vi "tfH12.vi"(0 "Resp1":dbl[](array[numeric]), 2 "采样率":i32, 4 "Resp2":dbl[](array[numeric])) -> (5 "ff":dbl[](array[numeric]), 6 "H12":cdb[](array[numeric]))   [LabVIEW 2018]
uses:
  <vilib>/Analysis/3filter.llb/Savitzky-Golay Filter (DBL).vi
  <vilib>/Analysis/NI_AALPro.lvlib
  <vilib>/Analysis/2dsp.llb/Real FFT.vi
  <vilib>/Analysis/NI_AALBase.lvlib
  <vilib>/Analysis/Matrix/NI_Matrix.lvlib
  <vilib>/Analysis/Matrix/Numeric/Conversions/Array To Matrix - CA2.vi
  <vilib>/Analysis/Matrix/Numeric/Conversions/Matrix To Array - CM.vi
  <vilib>/Analysis/baseanly.llb/Mean (CDB).vi
  <vilib>/Analysis/4window.llb/Hanning Window (DBL).vi
  <vilib>/ptbypt/NI_PtbyPt.lvlib
  <vilib>/measure/NI_MAPro.lvlib
  <vilib>/Analysis/4window.llb/windowTd.ctl
  <vilib>/measure/maspectr.llb/Frequency Response Function (Real-Im) 1-1.vi
  <vilib>/Analysis/3filter.llb/Savitzky-Golay Filter (CDB).vi
panel:
  out "averages completed":dbl
  out "unit label":string=" rms"
  out "IM":cluster{"X":dbl, "Y":dbl}[](graph)
  out "RE":cluster{"X":dbl, "Y":dbl}[](graph)
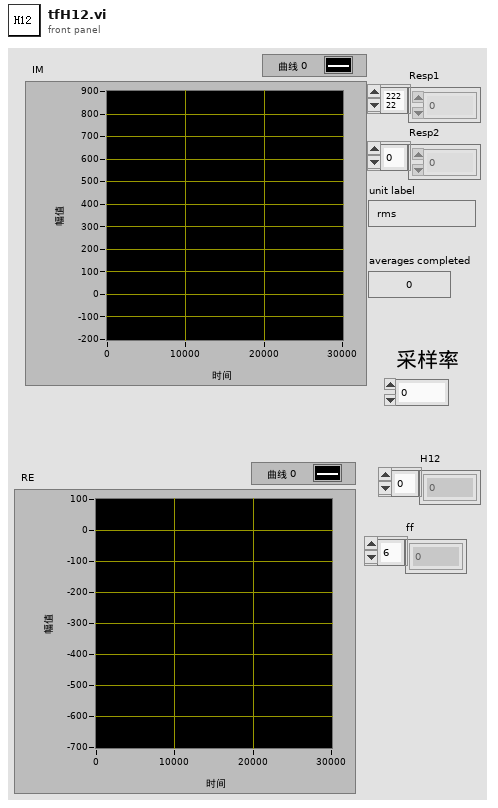
[diagram p1: front panel]
types:
  T1 = cluster{"averaging mode":enum16{"No averaging", "Vector averaging", "RMS averaging", "Peak hold"}, "weighting mode":enum16{"Linear", "Exponential"}, "number of averages":u32, "linear mode":enum16{"One shot", "Auto restart"}}
  T2 = cluster{"frequency range":cluster{"start frequency":dbl, "stop frequency":dbl}, "window":u16, "number of lines":i32, "% overlap":dbl}
  T3 = cluster{"averaging mode":enum16{"No averaging", "Vector averaging", "RMS averaging", "Peak hold"}, "weighting mode":enum16{"Linear", "Exponential"}, "number of averages":u32}
  T4 = typedef "NI_AALPro.lvlib/windowTd.ctl" = u32
  T5 = cluster{"f0":dbl, "df":dbl, "imaginary part":dbl[]}
  T6 = typedef "NI_Matrix.lvlib/ComplexMatrix.ctl" = cdb[][]
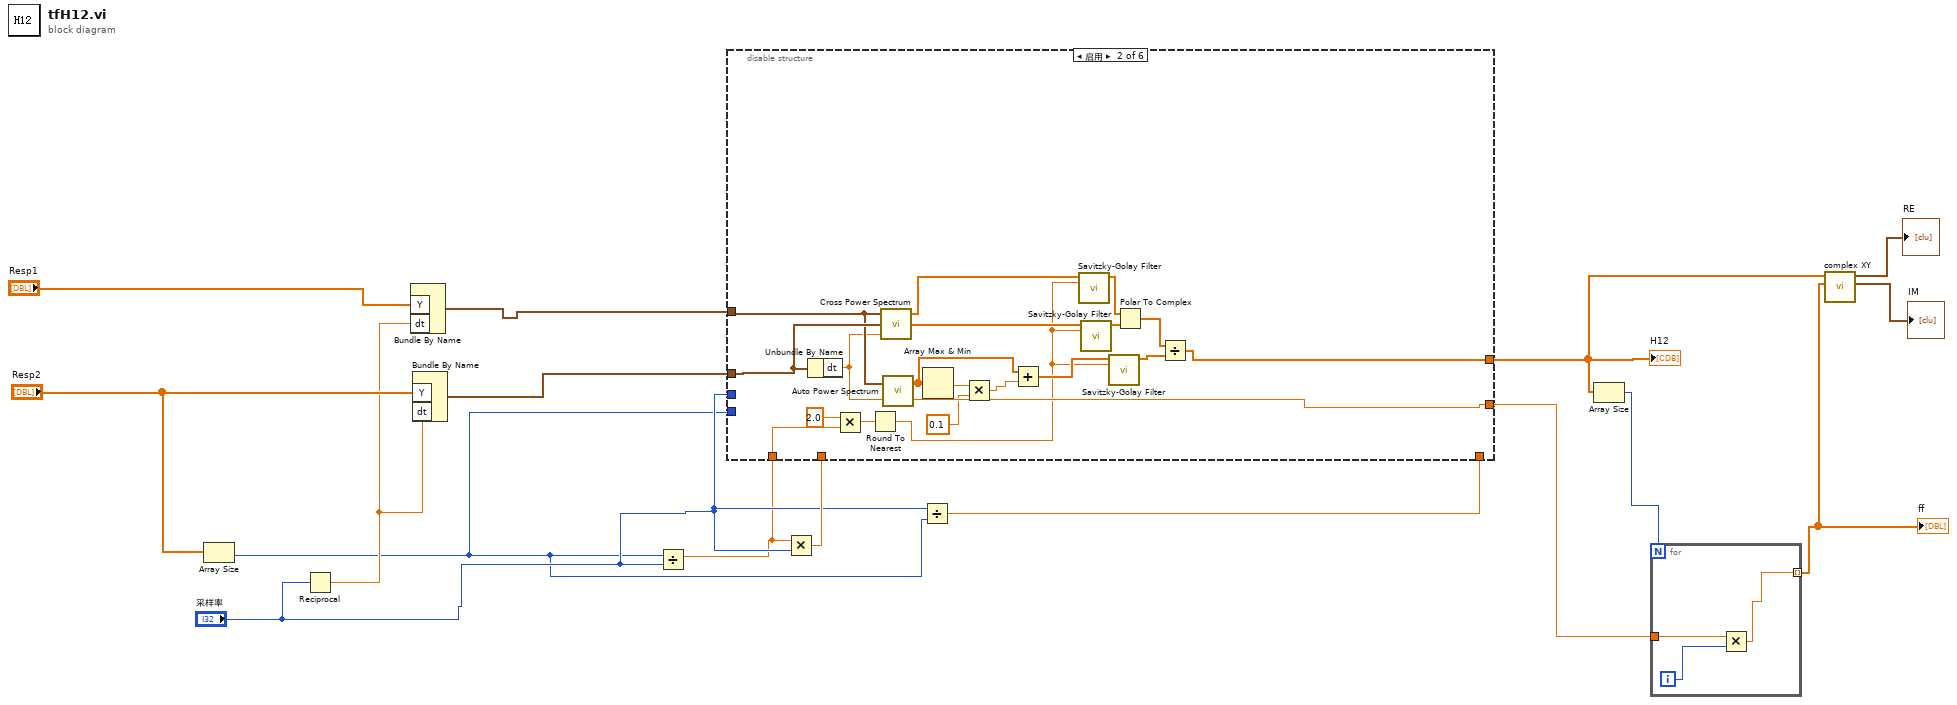
[diagram p0: block diagram]
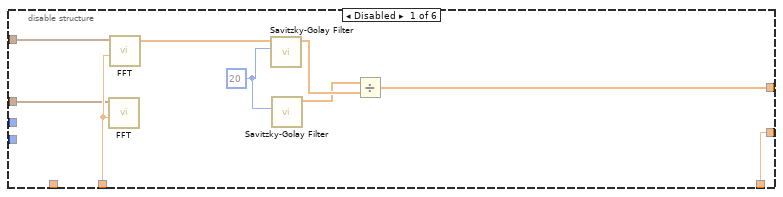
[diagram p2: hidden frame]
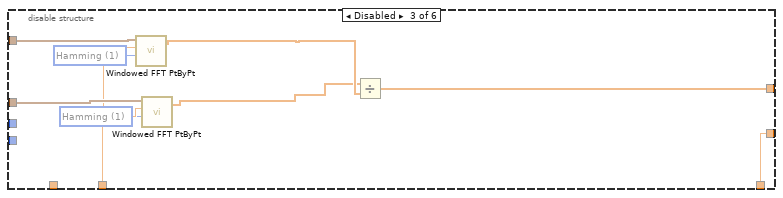
[diagram p3: hidden frame]
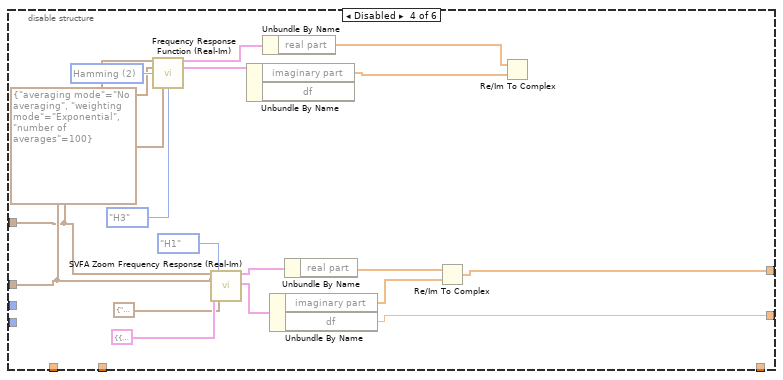
[diagram p4: hidden frame]
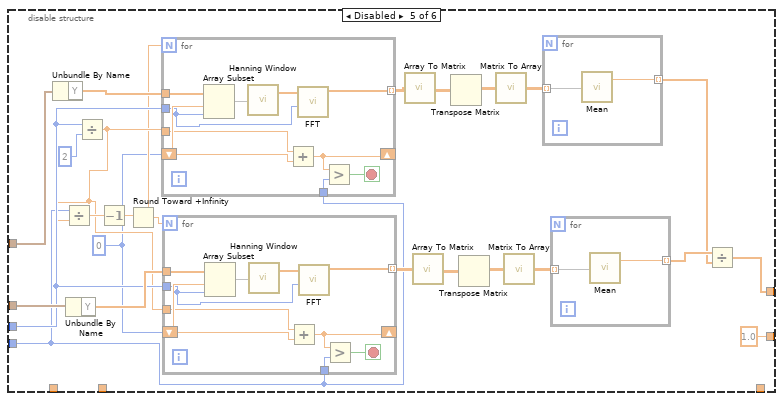
[diagram p5: hidden frame]
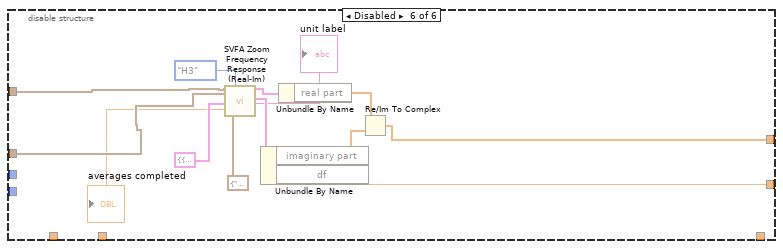
[diagram p6: hidden frame]
diagram:
  n1 = Array Size(array="Resp2") -> (size(s)=w6:i32)
  n2 = Reciprocal(x="采样率") -> (1/x=w12:dbl)
  n3 = Bundle By Name("Y"="Resp1", "dt"=w12) -> (w4:waveform(dbl))  [unwired: 1 in]
  n4 = Bundle By Name("Y"="Resp2", "dt"=w12) -> (w3:waveform(dbl))  [unwired: 1 in]
  n5 = Divide(x=w6, y="采样率") -> (x/y=w1:dbl)
  n6 = Multiply(x=w1, y="采样率") -> (x*y=w14:dbl)
  n7 = Divide(x="采样率", y=w6) -> (x/y=w5:dbl)
  n8 = disable-structure shown="启用" {
    disable-tunnel: [w25 w40 w54 w56 w80 w133] -> w2
    disable-tunnel: w14 -> [w24 _ w48 _ _ _]
    disable-tunnel: w3 -> [w23 w45 w50 w65 w79 w127]
    disable-tunnel: w4 -> [w22 w44 w52 w64 w96 w126]
    disable-tunnel: [w21 w42 w53 w55 1.0 w130] -> w11
    disable-tunnel: "采样率" -> [_ _ _ _ w77 _]
    disable-tunnel: w6 -> [_ _ _ _ w74 _]
    disable-tunnel: w5 -> [w21 _ w53 _ _ _]
    disable-tunnel: w1 -> [_ w29 _ _ _ _]
    frame Disabled {
      w19 = 20 ("side points")
      n9 = call-poly <vilib>:"FFT.vi"("FFT size"=w24, "X"=w23) -> ()  [unwired: 8 in, 2 out]
      n10 = call-poly <vilib>:"FFT.vi"("FFT size"=w24, "X"=w22) -> ("FFT {X}"=w20:cdb[])  [unwired: 8 in, 1 out]
      n11 = call-poly <vilib>:"Savitzky-Golay Filter.vi"("side points"=w19, "X"=w20) -> ("Filtered X"=w18:cdb[])  [unwired: 8 in, 1 out]
      n12 = call-poly <vilib>:"Savitzky-Golay Filter.vi"("side points"=w19) -> ("Filtered X"=w17:dbl[])  [unwired: 9 in, 1 out]
      n13 = Divide(x=w17, y=w18) -> (x/y=w25:cdb[])
    }
    frame Enabled {
      n14 = Unbundle By Name(w45) -> ("dt"=w43:dbl)
      n15 = Multiply(x=2.0, y=w29) -> (x*y=w27:dbl)
      n16 = Round To Nearest(number=w27) -> (nearest integer value=w26:dbl)
      n17 = call <vilib>:"Cross Power Spectrum.vi"("dt"=w43, "Signal Y (V)"=w45, "Signal X (V)"=w44) -> ("Cross Power XY Spectrum Phase (radians)"=w36:dbl[], "Cross Power XY Spectrum Mag (V^2rms)"=w38:dbl[])  [unwired: 1 out]
      n18 = call <vilib>:"Auto Power Spectrum.vi"("dt"=w43, "Signal (V)"=w44) -> ("df"=w42:dbl, "Power Spectrum (V^2 rms)"=w30:dbl[])
      n19 = Array Max & Min(array=w30) -> (min value=w34:dbl)  [unwired: 3 out]
      n20 = Multiply(x=w34, y=0.1) -> (x*y=w32:dbl)
      n21 = Add(x=w30, y=w32) -> (x+y=w31:dbl[])
      n22 = call-poly <vilib>:"Savitzky-Golay Filter.vi"("side points"=w26, "X"=w38) -> ("Filtered X"=w37:dbl[])  [unwired: 8 in, 1 out]
      n23 = call-poly <vilib>:"Savitzky-Golay Filter.vi"("side points"=w26, "X"=w36) -> ("Filtered X"=w35:dbl[])  [unwired: 8 in, 1 out]
      n24 = call-poly <vilib>:"Savitzky-Golay Filter.vi"("side points"=w26, "X"=w31) -> ("Filtered X"=w39:dbl[])  [unwired: 8 in, 1 out]
      n25 = Polar To Complex(1:w35, 2:w37) -> (0:w41:cdb[])
      n26 = Divide(x=w41, y=w39) -> (x/y=w40:cdb[])
    }
    frame Disabled {
      w46 = 1 items=["Hanning", "Hamming", "Blackman", "Exact Blackman", "Blackman-Harris"] ("window selector")
      w47 = 1 items=["Hanning", "Hamming", "Blackman", "Exact Blackman", "Blackman-Harris"] ("window selector")
      n27 = call <vilib>:"Windowed FFT PtByPt.vi"("x"=w52, "sample length"=w48, "window selector"=w46) -> ("Windowed FFT"=w51:cdb[])  [unwired: 2 in, 1 out]
      n28 = call <vilib>:"Windowed FFT PtByPt.vi"("x"=w50, "sample length"=w48, "window selector"=w47) -> ("Windowed FFT"=w49:cdb[])  [unwired: 2 in, 1 out]
      n29 = Divide(x=w49, y=w51) -> (x/y=w54:cdb[])
    }
    frame Disabled {
      w72 = T4 2 items=["矩形"=0, "Hanning"=1, "Hamming"=2, "Blackman-Harris"=3, "Exact Blackman"=4, "Blackman"=5, "Flat Top"=6, "4阶Blackman-Harris "=7, "7阶Blackman-Harris"=8, "Low Sidelobe"=9, "Blackman Nuttall"=11, "三角"=30, "Bartlett-Hanning"=31, "Bohman"=32, "Parzen"=33, "Welch"=34, "Kaiser"=60, "Dolph-Chebyshev"=61, "高斯"=62] ("window")
      n30 = call-poly <vilib>:"Frequency Response Function (Real-Im).vi"("time signal X"=w64, "time signal Y"=w65, "window"=w72, "averaging parameters"=T3 {"averaging mode"=enum."No averaging", "weighting mode"=enum."Exponential", "number of averages"=100}, "FRF Mode"=enum16{"H1", "H2", "H3"}."H3") -> ("real part"=w69:cluster{"f0":dbl, "df":dbl, "real part":dbl[]}, "imaginary part"=w71:T5)  [unwired: 5 in, 4 out]
      n31 = call <vilib>:"SVFA Zoom Frequency Response (Real-Im).vi"("stimulus signal X [EUx]"=w64, "response signal Y [EUy]"=w65, "zoom settings"=T2 {"frequency range"={"start frequency"=1.0, "stop frequency"=22050.0}, "window"=2, "number of lines"=22050, "% overlap"=50.0}, "FRF mode"=enum16{"H1", "H2", "H3"}."H1", "averaging parameters"=T1 {"averaging mode"=enum."No averaging", "weighting mode"=enum."Exponential", "number of averages"=10, "linear mode"=enum."Auto restart"}) -> ("real part [EUy/EUx rms]"=w61:cluster{"f0":dbl, "df":dbl, "real part":dbl[]}, "imaginary part [EUy/EUx rms]"=w60:T5)  [unwired: 6 in, 7 out]
      n32 = Unbundle By Name(w71) -> ("imaginary part"=w70:dbl[])  [unwired: 1 out]
      n33 = Unbundle By Name(w69) -> ("real part"=w68:dbl[])
      n34 = Unbundle By Name(w60) -> ("imaginary part"=w57:dbl[], "df"=w55:dbl)
      n35 = Unbundle By Name(w61) -> ("real part"=w58:dbl[])
      n36 = Re/Im To Complex(1:w57, 2:w58) -> (0:w56:cdb[])
      n37 = Re/Im To Complex(1:w70, 2:w68) -> ()  [unwired: 1 out]
    }
    frame Disabled {
      w73 = 0
      n38 = Unbundle By Name(w96) -> ("Y"=w95:dbl[])
      n39 = Unbundle By Name(w79) -> ("Y"=w78:dbl[])
      n40 = Divide(x=w77, y=2) -> (x/y=w76:dbl)
      n41 = Divide(x=w74, y=w76) -> (x/y=w89:dbl)
      n42 = Decrement(x=w89) -> (x-1=w88:dbl)
      n43 = Round Toward +Infinity(x=w88) -> (ceil(x): smallest int >= x=w75:dbl)
      n44 = for {
        N: w75 -> [_]
        tunnel: w77 -> [w113]
        shift-right: [w118] -> _
        shift-left: w73 -> [w119]
        tunnel: w95 -> [w120]
        tunnel: w74 -> [w117]
        tunnel: [w112] -> w94 mode=indexing
        tunnel: w76 -> [w111]
        stop <- w116 stop-if-true
        n45 = Array Subset(array=w120, index=w119, length=w113) -> (w115:dbl[])
        n46 = call-poly <vilib>:"Hanning Window.vi"("X"=w115) -> ("Windowed X"=w114:dbl[])  [unwired: 1 out]
        n47 = Add(x=w111, y=w119) -> (x+y=w118:dbl)
        n48 = call-poly <vilib>:"FFT.vi"("FFT size"=w113, "X"=w114) -> ("FFT {X}"=w112:cdb[])  [unwired: 8 in, 1 out]
        n49 = Greater?(x=w118, y=w117) -> (0:w116:bool)
      }
      n50 = for {
        N: w75 -> [_]
        tunnel: w77 -> [w101]
        shift-right: [w106] -> _
        shift-left: w73 -> [w107]
        tunnel: w78 -> [w108]
        tunnel: w74 -> [w105]
        tunnel: [w100] -> w83 mode=indexing
        tunnel: w76 -> [w99]
        stop <- w104 stop-if-true
        n51 = Array Subset(array=w108, index=w107, length=w101) -> (w103:dbl[])
        n52 = call-poly <vilib>:"Hanning Window.vi"("X"=w103) -> ("Windowed X"=w102:dbl[])  [unwired: 1 out]
        n53 = Add(x=w99, y=w107) -> (x+y=w106:dbl)
        n54 = call-poly <vilib>:"FFT.vi"("FFT size"=w101, "X"=w102) -> ("FFT {X}"=w100:cdb[])  [unwired: 8 in, 1 out]
        n55 = Greater?(x=w106, y=w105) -> (0:w104:bool)
      }
      n56 = call-poly <vilib>:"Array To Matrix.vi"("Complex 2D Array"=w94) -> ("Complex Matrix"=w93:T6)
      n57 = call-poly <vilib>:"Array To Matrix.vi"("Complex 2D Array"=w83) -> ("Complex Matrix"=w84:T6)
      n58 = Transpose Matrix(1:w93) -> (0:w92:T6)
      n59 = Transpose Matrix(1:w84) -> (0:w85:T6)
      n60 = call-poly <vilib>:"Matrix To Array.vi"("Complex Matrix"=w92) -> ("Complex 2D Array"=w91:cdb[][])
      n61 = call-poly <vilib>:"Matrix To Array.vi"("Complex Matrix"=w85) -> ("Complex 2D Array"=w86:cdb[][])
      n62 = for {
        tunnel: w91 -> [w110] mode=indexing
        tunnel: [w109] -> w81 mode=indexing
        n63 = call-poly <vilib>:"Mean.vi"("X"=w110) -> ("mean"=w109:cdb)  [unwired: 1 out]
      }
      n64 = for {
        tunnel: w86 -> [w98] mode=indexing
        tunnel: [w97] -> w82 mode=indexing
        n65 = call-poly <vilib>:"Mean.vi"("X"=w98) -> ("mean"=w97:cdb)  [unwired: 1 out]
      }
      n66 = Divide(x=w82, y=w81) -> (x/y=w80:cdb[])
    }
    frame Disabled {
      n67 = call <vilib>:"SVFA Zoom Frequency Response (Real-Im).vi"("stimulus signal X [EUx]"=w126, "response signal Y [EUy]"=w127, "zoom settings"=T2 {"frequency range"={"start frequency"=137.0, "stop frequency"=6198.0}, "window"=1, "number of lines"=6062, "% overlap"=50.0}, "FRF mode"=enum16{"H1", "H2", "H3"}."H3", "averaging parameters"=T1 {"averaging mode"=enum."Vector averaging", "weighting mode"=enum."Linear", "number of averages"=22050, "linear mode"=enum."One shot"}) -> ("averages completed"=→"averages completed":dbl, "real part [EUy/EUx rms]"=w129:cluster{"f0":dbl, "df":dbl, "real part":dbl[]}, "imaginary part [EUy/EUx rms]"=w128:T5, "unit label"=→"unit label":string)  [unwired: 6 in, 5 out]
      n68 = Unbundle By Name(w128) -> ("imaginary part"=w131:dbl[], "df"=w130:dbl)
      n69 = Unbundle By Name(w129) -> ("real part"=w132:dbl[])
      n70 = Re/Im To Complex(1:w131, 2:w132) -> (0:w133:cdb[])
    }
  }
  "H12" <- w2
  n71 = Array Size(array=w2) -> (size(s)=w16:i32)
  n72 = for {
    N: w16 -> [_]
    tunnel: w11 -> [w136]
    tunnel: [w134] -> w10 mode=indexing
    i -> [w135]
    n73 = Multiply(x=w136, y=w135) -> (x*y=w134:dbl)
  }
  "ff" <- w10
  n74 = call "complex XY.vi"("f"=w10, "数组"=w2) -> ("IM"=→"IM":cluster{"X":dbl, "Y":dbl}[], "RE"=→"RE":cluster{"X":dbl, "Y":dbl}[])  [unwired: 8 in]
